vi "Read Example Test 1.vi"() -> ()   [LabVIEW 2014]
panel:
  out "__return":string
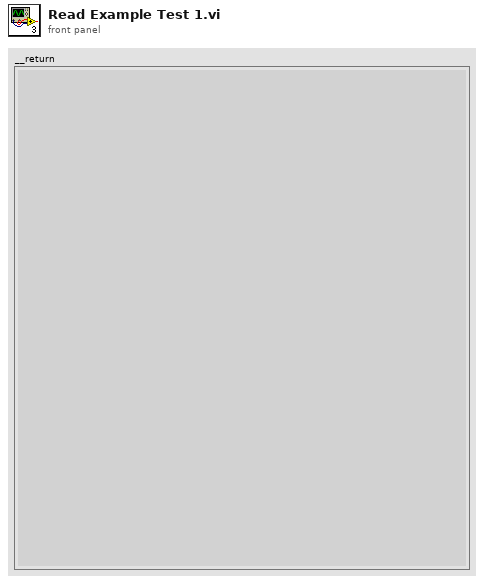
[diagram p1: front panel]
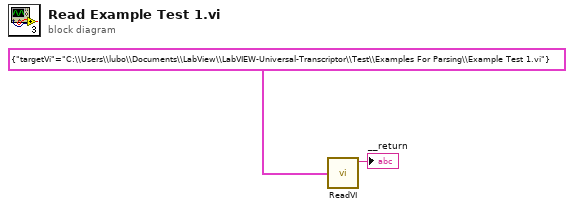
[diagram p0: block diagram]
diagram:
  n1 = call "ReadVI.vi"("__args"=cluster{"targetVi":string} {"targetVi"="C:\\Users\\lubo\\Documents\\LabView\\LabVIEW-Universal-Transcriptor\\Test\\Examples For Parsing\\Example Test 1.vi"}) -> ("__return"=→"__return":string)  [unwired: 3 out]
